vi "ADC_GetConfig.vi"(8 "error in (no error)":errorcluster, 11 "DeviceIndex":u32 format="%08x") -> (0 "error out":errorcluster {"code" format="%.0x"}, 1 "ConfigBufSize":u32, 3 "pConfigBuf":u8[](array[numeric]))   [LabVIEW 2012]
doc: "unsigned long ADC_GetConfig(\nunsigned long DeviceIndex - number from 0-31 indicating from which device you wish to get the\nA/D configuration\nunsigned char *pConfigBuf - a pointer to the first of an array of bytes for configuration data\nunsigned long *ConfigBufSize - a pointer to a variable holding the number of configuration bytes\nto read. Will be set to the number of configuration"
uses:
  Windows/System32/AIOUSB.dll
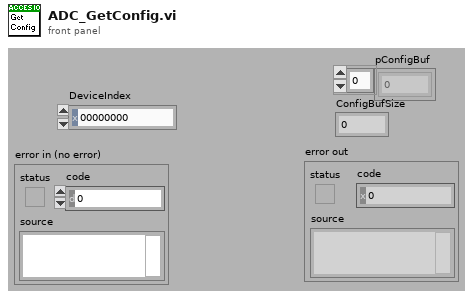
[diagram p1: front panel]
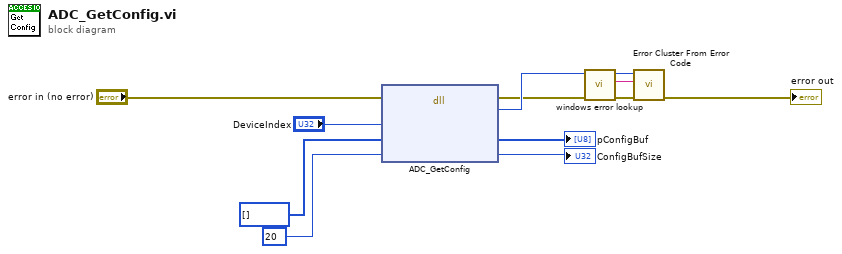
[diagram p0: block diagram]
diagram:
  n1 = dll-call lib="C:/Windows/System32/AIOUSB.dll" fn="ADC_GetConfig"(error in="error in (no error)", "DeviceIndex"="DeviceIndex", "pConfigBuf"=u8[] [], "ConfigBufSize"=u32 20) -> (error out=w2:errorcluster, "return type"=w3:u32, "pConfigBuf"=→"pConfigBuf":u8[], "ConfigBufSize"=→"ConfigBufSize":u32)  [unwired: 3 in, 1 out]
  n2 = call "windows error lookup.vi"("error in (no error)"=w2, "Error Code"=w3) -> ("error out"=w1:errorcluster, "error message (\"\")"=w5:string)  [unwired: 8 in]
  n3 = call <vilib>:"Error Cluster From Error Code.vi"("error in (no error)"=w1, "error message (\"\")"=w5, "error code (0)"=w3) -> ("error out"=→"error out":errorcluster)  [unwired: 6 in]
